vi "LT_set_remote_cont.vi"(7 "remote_cont":bool, 8 "error in":errorcluster, 10 "dev_param_in":T1={"Length of data block (14)"=14, "Converter address (0)"=0, "Converter type\n(180: Turbovac 350/450 i)"=180, "PZD1 STW, ZSW (0)"=0, "PZD2 HSW, HIW (0)"=0} {"Converter type\n(180: Turbovac 350/450 i)" items=["Turbovac 350/450 i"=180, "Turbovac 350/450 i with optional interface"=181, "Turbovac 350/450 iX"=182, "Turbovac  90/250 i"=190, "Turbovac  90/250 with optional interface"=191, "Turbovac  90/250 iX"=192, "Turbovac  850/950 i"=195, "Turbovac  850/950 i with optional interface"=196, "Turbovac  850/950 iX"=197, "Turbovac 1350/1450 i"=185, "Turbovac 1350/1450 i with optional interface"=186, "Turbovac 1350/1450 iX"=187]; "Length of data block (14)" items=["14"=14, "22"=22]}, 11 "VISA in":refnum<visa-resource-name>="COM43") -> (0 "error out":errorcluster, 2 "dev_param_out":T3={"Length of data block"=14, "Converter address"=0, "Converter type"=180, "PZD1"=0, "PZD2"=0} {"Converter type" items=["Turbovac 350/450 i"=180, "Turbovac 350/450 i with optional interface"=181, "Turbovac 350/450 iX"=182, "Turbovac  90/250 i"=190, "Turbovac  90/250 with optional interface"=191, "Turbovac  90/250 iX"=192, "Turbovac  850/950 i"=195, "Turbovac  850/950 i with optional interface"=196, "Turbovac  850/950 iX"=197, "Turbovac 1350/1450 i"=185, "Turbovac 1350/1450 i with optional interface"=186, "Turbovac 1350/1450 iX"=187]; "Length of data block" items=["14"=14, "22"=22]}, 3 "VISA out":refnum<visa-resource-name>, 4 "status":bool)   [LabVIEW 2019]
doc: "Example VI to demonstrate the use of the Oerlikon Leybold TMP driver."
uses:
  <instrlib>/Leybold TURBOVAC/Public/Ctl/Device Parameters Indicator.ctl
  <instrlib>/Leybold TURBOVAC/Public/Ctl/Converter Type Indicator.ctl
  <instrlib>/Leybold TURBOVAC/Public/Ctl/Device Parameters Control.ctl
  <instrlib>/Leybold TURBOVAC/Public/Ctl/Converter Type Control.ctl
  <instrlib>/Leybold TURBOVAC/Leybold TURBOVAC.lvlib
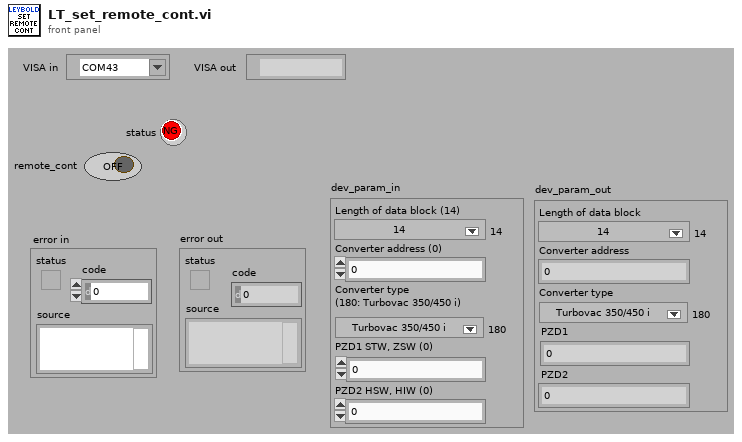
[diagram p1: front panel]
types:
  T1 = typedef "Leybold TURBOVAC.lvlib/Device Parameters Control.ctl" = cluster{"Length of data block (14)":u8, "Converter address (0)":u8, "Converter type\n(180: Turbovac 350/450 i)":T2, "PZD1 STW, ZSW (0)":u16, "PZD2 HSW, HIW (0)":u16}
  T2 = typedef "Leybold TURBOVAC.lvlib/Converter Type Control.ctl" = u16
  T3 = typedef "Leybold TURBOVAC.lvlib/Device Parameters Indicator.ctl" = cluster{"Length of data block":u8, "Converter address":u8, "Converter type":T4, "PZD1":u16, "PZD2":u16}
  T4 = typedef "Leybold TURBOVAC.lvlib/Converter Type Indicator.ctl" = u16
  T5 = cluster{"Ready to switch on":bool, "Ignore":bool, "Operation enabled":bool, "Fault condition is active":bool, "Pump speed is increasing":bool, "Pump speed is decreasing":bool, "Switch on lock":bool, "Warning temperature":bool, "Ignore":bool, "Frequency converter accepts parameters":bool, "Normal operation":bool, "Pump is revolving":bool, "Ignore":bool, "Warning overload":bool, "Collective warning":bool, "Remote has been activated":bool}
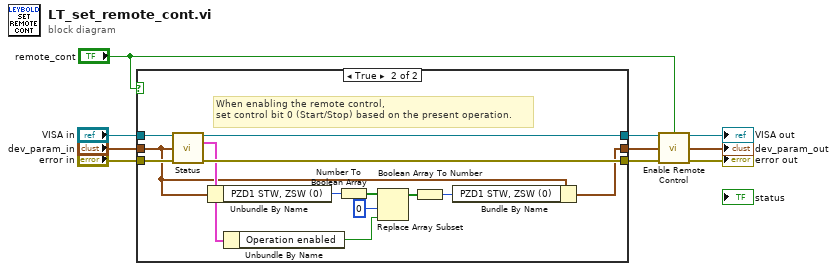
[diagram p0: block diagram]
diagram:
  n1 = case shown="True" "remote_cont" {
    tunnel: [w13 w26] -> w10
    tunnel: [w11 w25] -> w9
    tunnel: [w12 w14] -> w8
    tunnel: "VISA in" -> [w13 w24]
    tunnel: "error in" -> [w11 w23]
    tunnel: "dev_param_in" -> [w12 w15]
    frame False {
    }
    frame True {
      # "When enabling the remote control,\nset control bit 0 (Start/Stop) based on the present operation."
      n2 = call <instrlib>:"Status.vi"("VISA resource name"=w24, "Device parameters"=w15, "error in (no error)"=w23) -> ("VISA resource name out"=w26:refnum<visa-resource-name>, "Status word"=w22:T5, "error out"=w25:errorcluster)  [unwired: 8 in, 2 out]
      n3 = Unbundle By Name(w15) -> ("PZD1 STW, ZSW (0)"=w17:u16)
      n4 = Unbundle By Name(w22) -> ("Operation enabled"=w16:bool)
      n5 = Number To Boolean Array(number=w17) -> (Boolean array=w21:bool[])
      n6 = Replace Array Subset(array=w21, new element=w16, index=0) -> (w20:bool[])
      n7 = Boolean Array To Number(Boolean array=w20) -> (number=w19:u32)
      n8 = Bundle By Name(cluster=w15, "PZD1 STW, ZSW (0)"=w19) -> (w14:T1)
    }
  }
  n9 = call <instrlib>:"Enable Remote Control.vi"("VISA resource name"=w10, "Enable Remote Control (F: off)"="remote_cont", "Device parameters"=w8, "error in (no error)"=w9) -> ("VISA resource name out"=→"VISA out":refnum<visa-resource-name>, "Device parameters out"=→"dev_param_out":T3, "error out"=→"error out":errorcluster)  [unwired: 9 in]
